vi "ValveToDAQPort.vi"(1 "Valves":bool[](array[boolean])) -> (0 "DAQ Ports":bool[](array[boolean]))   [LabVIEW 2022 SP3]
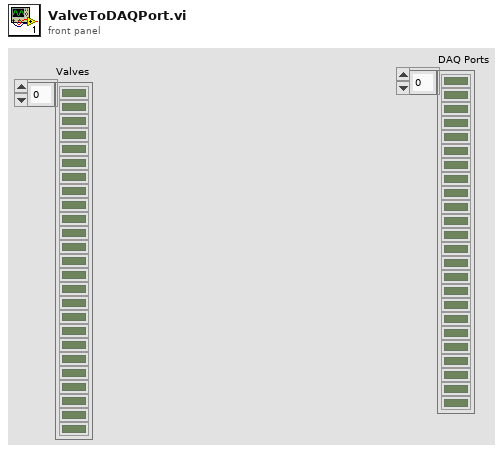
[diagram p1: front panel]
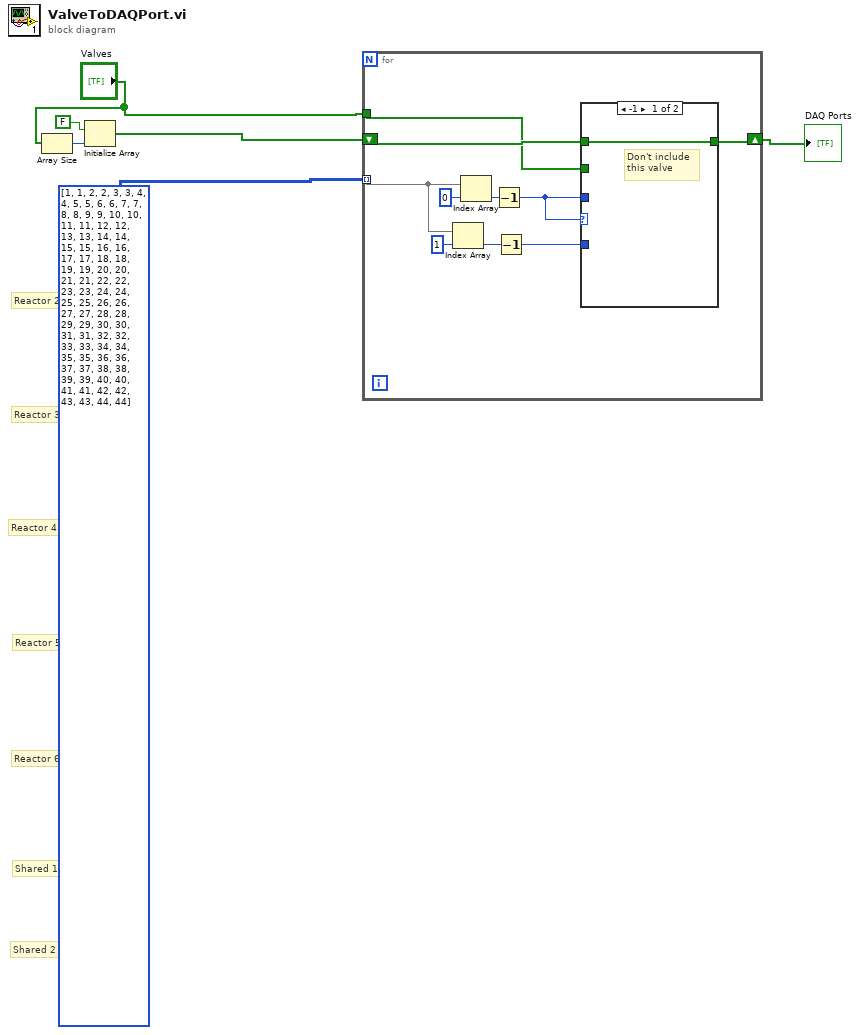
[diagram p0: block diagram]
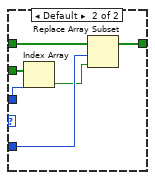
[diagram p2: hidden frame]
diagram:
  # "Shared 2 -->"
  # "Shared 1 -->"
  # "Reactor 6 -->"
  # "Reactor 5 -->"
  # "Reactor 4 -->"
  # "Reactor 3 -->"
  # "Reactor 2 -->"
  n1 = Array Size(array="Valves") -> (size(s)=w2:i32)
  n2 = Initialize Array(FALSE, w2) -> (w4:bool[])
  n3 = for {
    tunnel: i32[][] [[1, 1], [2, 2], [3, 3], [4, 4], [5, 5], [6, 6], [7, 7], [8, 8], [9, 9], [10, 10], [11, 11], [12, 12], [13, 13], [14, 14], [15, 15], [16, 16], [17, 17], [18, 18], [19, 19], [20, 20], [21, 21], [22, 22], [23, 23], [24, 24], [25, 25], [26, 26], [27, 27], [28, 28], [29, 29], [30, 30], [31, 31], [32, 32], [33, 33], [34, 34], [35, 35], [36, 36], [37, 37], [38, 38], [39, 39], [40, 40], [41, 41], [42, 42], [43, 43], [44, 44]] -> [w12] mode=indexing
    tunnel: "Valves" -> [w13]
    shift-right: [w8] -> w3
    shift-left: w4 -> [w16]
    n4 = Index Array(array=w12, index=1) -> (element=w10:i32)
    n5 = Index Array(array=w12, index=0) -> (element=w14:i32)
    n6 = Decrement(x=w14) -> (x-1=w7:i32)
    n7 = Decrement(x=w10) -> (x-1=w9:i32)
    n8 = case shown="-1" w7 {
      tunnel: w16 -> [w17 w23]
      tunnel: w7 -> [_ w22]
      tunnel: w13 -> [_ w21]
      tunnel: w9 -> [_ w20]
      tunnel: [w17 w18] -> w8
      frame -1 {
        # "Don't include\nthis valve"
      }
      frame Default {
        n9 = Index Array(array=w21, index=w22) -> (element=w19:bool)
        n10 = Replace Array Subset(array=w23, new element=w19, index=w20) -> (w18:bool[])
      }
    }
  }
  "DAQ Ports" <- w3
